vi "comm wait for event.vi"(8 "error in (no error)":errorcluster, 10 "milliseconds timeout":u32, 11 "Comm Handle":u32) -> (0 "error out":errorcluster, 2 "event mask":u32, 3 "dup Comm Handle":u32)   [LabVIEW 2013, in "lvserial.lvlib"]
doc: "Waits for an event to occur for a specified communications device."
uses:
  lvserial.lvlib
  lvserial.dll
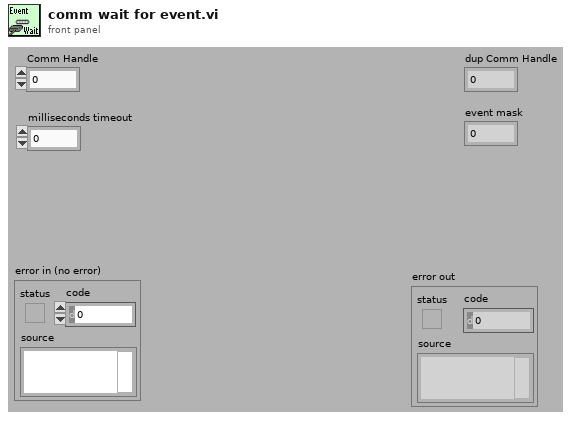
[diagram p1: front panel]
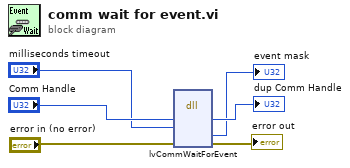
[diagram p0: block diagram]
diagram:
  n1 = dll-call lib="lvserial.dll" fn="lvCommWaitForEvent"("hComm"="Comm Handle", "ulTimeout"="milliseconds timeout", "error in (no error)"="error in (no error)") -> ("hComm"=→"dup Comm Handle":u32, "pulEventMask"=→"event mask":u32, "error in (no error)"=→"error out":errorcluster)  [unwired: 5 in, 3 out]
